vi "ACC GAIN CALCULATION.vi"(10 "AO Slop & Offset":sgl[](array[numeric]), 11 "AO Slop & Offset 2":sgl[](array[numeric])) -> (2 "E-Acc_1":T1, 3 "E-Acc_1 2":T1)   [LabVIEW 2018]
types:
  T1 = cluster{"Gain":fxp<+/-,20,5>, "OffSet":fxp<+/-,20,5>}
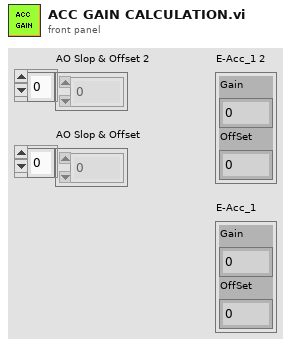
[diagram p1: front panel]
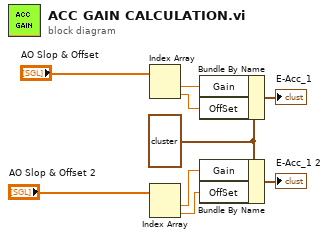
[diagram p0: block diagram]
diagram:
  w9 = T1 {"Gain"=0.0, "OffSet"=1.5} ("E-Acc_1")
  n1 = Index Array(array="AO Slop & Offset") -> (element #1=w5:sgl, element #2=w6:sgl)  [unwired: 2 in]
  n2 = Index Array(array="AO Slop & Offset 2") -> (element #1=w2:sgl, element #2=w3:sgl)  [unwired: 2 in]
  n3 = Bundle By Name(cluster=w9, "Gain"=w5, "OffSet"=w6) -> (→"E-Acc_1":T1)
  n4 = Bundle By Name(cluster=w9, "Gain"=w2, "OffSet"=w3) -> (→"E-Acc_1 2":T1)
